vi "StreamingVideoData.vi"(8 "error in (no error)":errorcluster, 11 "CameraDemo in":refnum<class "CameraDemo.lvclass">) -> (0 "error out":errorcluster, 3 "CameraDemo out":refnum<class "CameraDemo.lvclass">)   [LabVIEW 2020, in "CameraI2COUSB.lvlib" / "CameraDemo.lvclass"]
uses:
  CameraDemo.lvclass
  <vilib>/picture/picture.llb/imagedata.ctl
  CameraDemo.lvclass/CameraDemo.ctl
panel:
  in  "Stop":bool
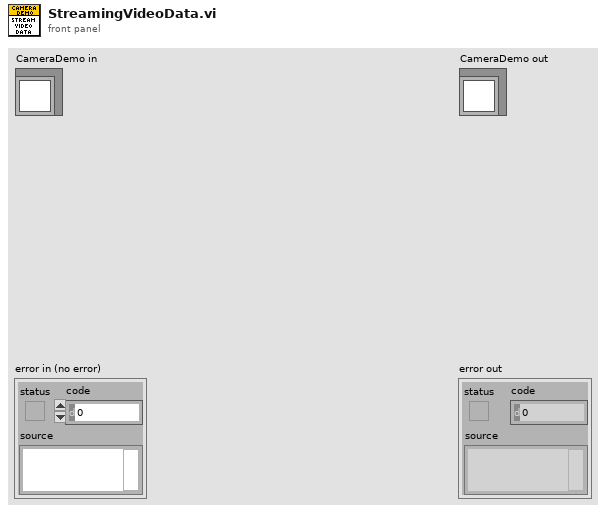
[diagram p1: front panel]
types:
  T1 = typedef "imagedata.ctl" = cluster{"image type":i32, "image depth":i32, "image":u8[], "mask":u8[], "colors":u32[], "Rectangle":cluster{"left":i16, "top":i16, "right":i16, "bottom":i16}}
  T2 = enum16{"Get Video Frame File Name", "Read Video Frames", "Signal Video Frame Data"}
  T3 = typedef "ICamera.lvlib/ICamera.lvclass/StreamDataEvent.ctl" = refnum<user-event>
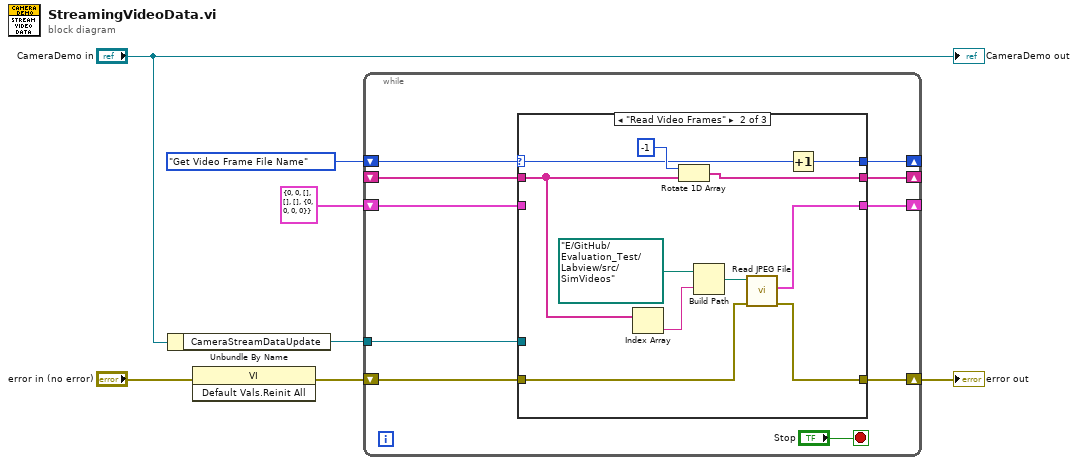
[diagram p0: block diagram]
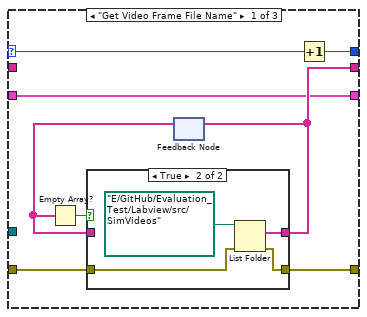
[diagram p2: hidden frame]
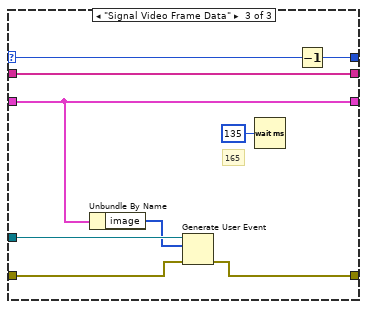
[diagram p4: hidden frame]
diagram:
  n1 = Unbundle By Name("CameraDemo in") -> ("CameraStreamDataUpdate"=w5:T3)
  n2 = invoke class="VI" method="Default Vals.Reinit All"(error in="error in (no error)") -> (error out=w4:errorcluster)  [unwired: 2 in, 2 out]
  n3 = while {
    shift-right: [w16] -> _
    shift-left: T2."Get Video Frame File Name" ("States") -> [w17]
    shift-right: [w15] -> _
    shift-left: _ -> [w14]
    shift-right: [w13] -> _
    shift-left: T1 {"image type"=0, "image depth"=0, "image"=[], "mask"=[], "colors"=[], "Rectangle"={"left"=0, "top"=0, "right"=0, "bottom"=0}} ("image data") -> [w12]
    tunnel: w5 -> [w10]
    shift-right: [w8] -> w1
    shift-left: w4 -> [w9]
    stop <- "Stop" stop-if-true
    n4 = case shown="\"Read Video Frames\"" w17 {
      selector: w17 -> [w23 w36 w51]
      tunnel: [w22 w37 w50] -> w16
      tunnel: [w21 w38 w49] -> w15
      tunnel: w14 -> [_ w39 w49]
      tunnel: [w20 w35 w46] -> w13
      tunnel: w12 -> [w20 _ w46]
      tunnel: w10 -> [_ _ w47]
      tunnel: w9 -> [w19 w33 w45]
      tunnel: [w18 w32 w43] -> w8
      frame "Get Video Frame File Name" {
        n5 = feedback #1() -> (w24:string[])  [unwired: 1 in]
        n6 = Empty Array?(array=w24) -> (empty?=w25:bool)
        n7 = case shown="True" w25 {
          tunnel: [w27 w30] -> w21
          tunnel: w24 -> [w27 _]
          tunnel: w19 -> [w26 w29]
          tunnel: [w26 w28] -> w18
          frame False {
          }
          frame True {
            n8 = List Folder(path=path "E:/GitHub/Evaluation_Test/Labview/src/SimVideos", error in=w29) -> (filenames=w30:string[], error out=w28:errorcluster)  [unwired: 2 in, 2 out]
          }
        }
        n9 = feedback-in #1(w21) -> ()
        n10 = Increment(x=w23) -> (x+1=w22:T2)
      }
      frame "Read Video Frames" {
        n11 = Index Array(array=w39) -> (element=w42:string)  [unwired: 1 in]
        n12 = Rotate 1D Array(1:w39, 2:-1 ("n")) -> (0:w38:string[])
        n13 = Build Path(base path=path "E:/GitHub/Evaluation_Test/Labview/src/SimVideos", name or relative path=w42) -> (appended path=w41:path)
        n14 = call <vilib>:"Read JPEG File.vi"("error in (no error)"=w33, "path to JPEG file"=w41) -> ("error out"=w32:errorcluster, "image data"=w35:T1)  [unwired: 7 in, 1 out]
        n15 = Increment(x=w36) -> (x+1=w37:T2)
      }
      frame "Signal Video Frame Data" {
        # "165"
        n16 = Unbundle By Name(w46) -> ("image"=w44:u8[])
        n17 = Generate User Event(user event=w47, event data cluster=w44, error in=w45) -> (error out=w43:errorcluster)  [unwired: 1 in, 1 out]
        n18 = Wait (ms)(milliseconds to wait=u32 135) -> ()  [unwired: 1 out]
        n19 = Decrement(x=w51) -> (x-1=w50:T2)
      }
    }
  }
  "error out" <- w1
  "CameraDemo out" <- "CameraDemo in"
